vi "Set Smooth Diff Window.vi"(8 "error in (no error)":errorcluster, 10 "Window":i32=10, 11 "MF3 in":refnum<class "MF3.lvclass">) -> (0 "error out":errorcluster, 3 "MF3 out":refnum<class "MF3.lvclass">)   [LabVIEW 2011, in "MF3.lvclass"]
uses:
  MF3.lvclass
  MF3.lvclass/MF3.ctl
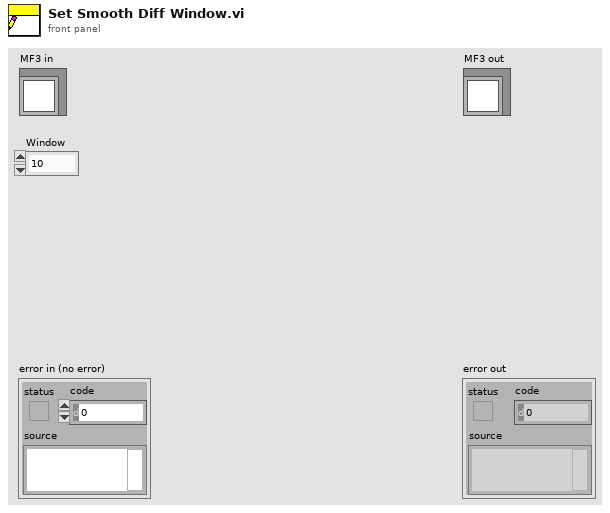
[diagram p1: front panel]
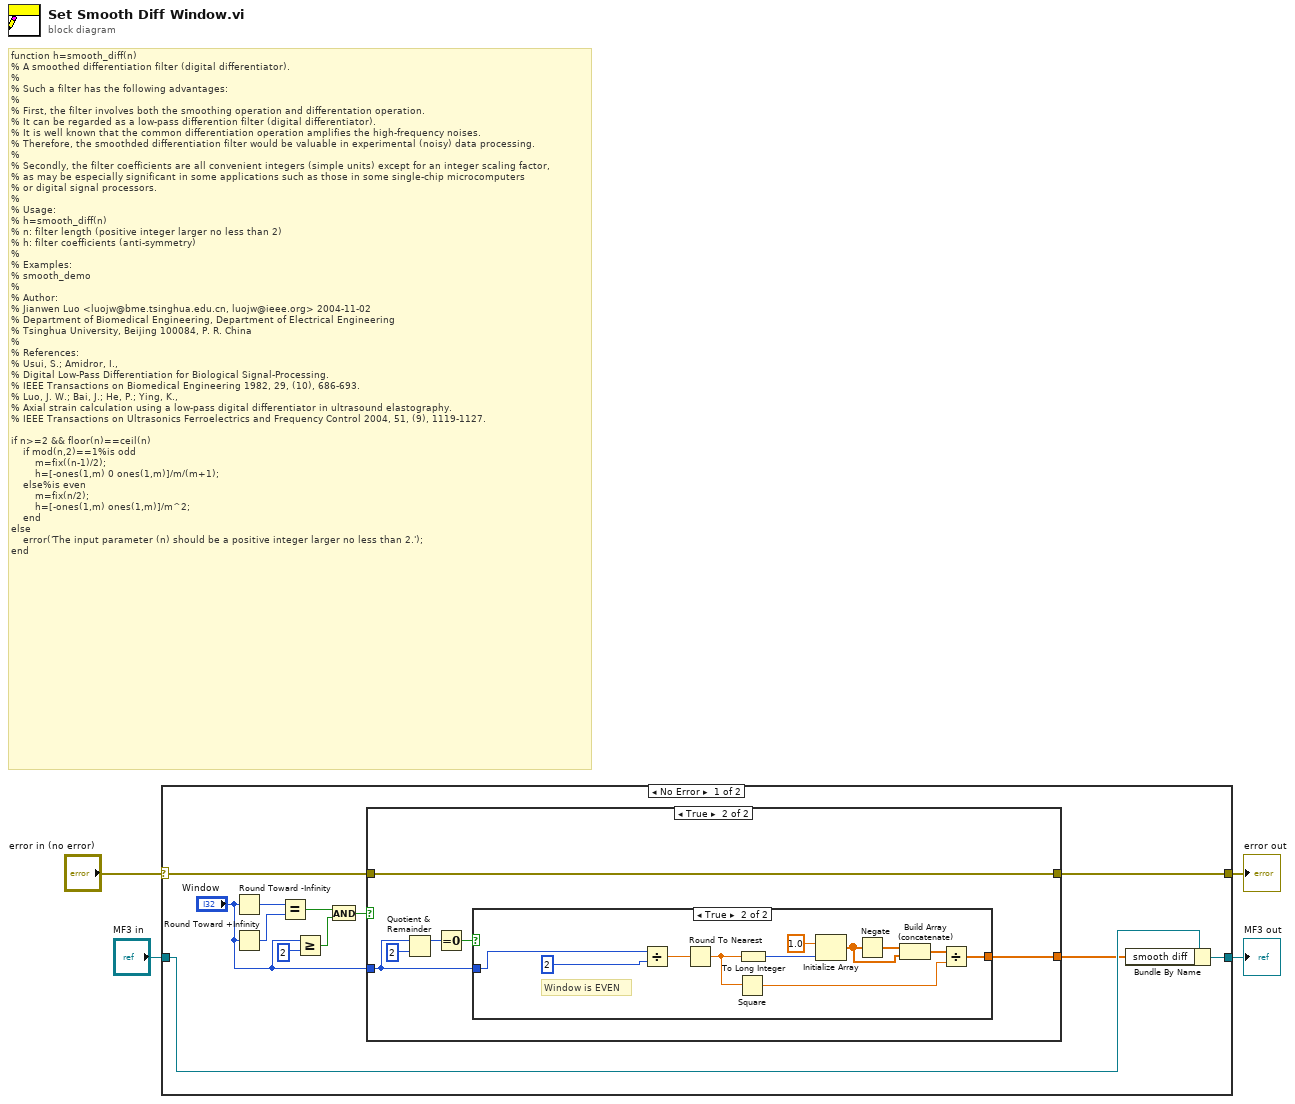
[diagram p0: block diagram]
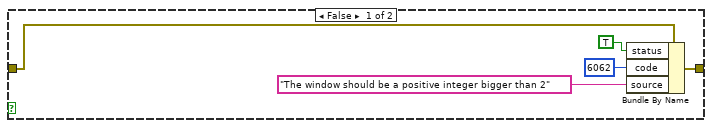
[diagram p2: hidden frame]
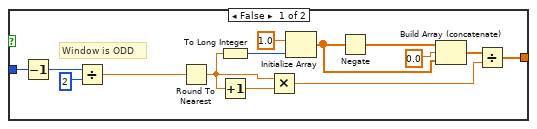
[diagram p3: hidden frame]
diagram:
  # "function h=smooth_diff(n)\n% A smoothed differentiation filter (digital differentiator). \n%\n% Such a filter has the following advantages:\n% \n% First, the filter involves both the smoothing operation and differentation operation. \n% It can be regarded as a low-pass differention filter (digital differentiator). \n% It is well known that the common differentiation operation amplifies the high-frequency noises.\n% Therefore, the smoothded differentiation filter would be valuable in experimental (noisy) data processing. \n% \n% Secondly, the filter coefficients are all convenient integers (simple units) except for an integer scaling factor,\n% as may be especially significant in some applications such as those in some single-chip microcomputers\n% or digital signal processors. \n% \n% Usage:\n% h=smooth_diff(n)\n% n: filter length (positive integer larger no less than 2)\n% h: filter coefficients (anti-symmetry)\n%\n% Examples:\n% smooth_demo\n%\n% Author:\n% Jianwen Luo <luojw@bme.tsinghua.edu.cn, luojw@ieee.org> 2004-11-02\n% Department of Biomedical Engineering, Department of Electrical Engineering\n% Tsinghua University, Beijing 100084, P. R. China  \n% \n% References:\n% Usui, S.; Amidror, I., \n% Digital Low-Pass Differentiation for Biological Signal-Processing. \n% IEEE Transactions on Biomedical Engineering 1982, 29, (10), 686-693.\n% Luo, J. W.; Bai, J.; He, P.; Ying, K., \n% Axial strain calculation using a low-pass digital differentiator in ultrasound elastography. \n% IEEE Transactions on Ultrasonics Ferroelectrics and Frequency Control 2004, 51, (9), 1119-1127.\n\nif n>=2 && floor(n)==ceil(n)\n    if mod(n,2)==1%is odd\n        m=fix((n-1)/2);\n        h=[-ones(1,m) 0 ones(1,m)]/m/(m+1);\n    else%is even\n        m=fix(n/2);\n        h=[-ones(1,m) ones(1,m)]/m^2;\n    end\nelse    \n    error('The input parameter (n) should be a positive integer larger no less than 2.');\nend"
  n1 = case shown="No Error" "error in (no error)" {
    selector: "error in (no error)" -> [w10 w53]
    tunnel: [w9 w53] -> w4
    tunnel: [w6 w54] -> w2
    tunnel: "MF3 in" -> [w7 w54]
    frame No Error {
      n2 = Round Toward -Infinity(1:"Window") -> (0:w12:i32)
      n3 = Round Toward +Infinity(x="Window") -> (ceil(x): smallest int >= x=w11:i32)
      n4 = Equal?(x=w12, y=w11) -> (x = y?=w13:bool)
      n5 = Greater Or Equal?(x="Window", y=2) -> (x >= y?=w15:bool)
      n6 = And(x=w13, y=w15) -> (x .and. y?=w16:bool)
      n7 = case shown="True" w16 {
        tunnel: [w21 w27] -> w9
        tunnel: w10 -> [w17 w27]
        tunnel: "Window" -> [_ w23]
        tunnel: [_ w22] -> w5
        frame False {
          n8 = Bundle By Name(cluster=w17, "status"=TRUE, "code"=6062, "source"="The window should be a positive integer bigger than 2") -> (w21:errorcluster)
        }
        frame True {
          n9 = Quotient & Remainder(x=w23, y=2) -> (x-y*floor(x/y)=w25:i32)  [unwired: 1 out]
          n10 = Equal To 0?(x=w25) -> (x = 0?=w24:bool)
          n11 = case shown="True" w24 {
            tunnel: w23 -> [w41 w47]
            tunnel: [w31 w45] -> w22
            frame False {
              # "Window is ODD"
              n12 = Decrement(x=w41) -> (x-1=w40:i32)
              n13 = Divide(x=w40, y=2) -> (x/y=w38:dbl)
              n14 = Round To Nearest(number=w38) -> (nearest integer value=w28:dbl)
              n15 = To Long Integer(number=w28) -> (32bit integer=w37:i32)
              n16 = Increment(x=w28) -> (x+1=w29:dbl)
              n17 = Multiply(x=w28, y=w29) -> (x*y=w30:dbl)
              n18 = Initialize Array(1.0 ("element"), w37) -> (w33:dbl[])
              n19 = Negate(x=w33) -> (-x=w35:dbl[])
              n20 = Build Array (concatenate)(w35, 0.0 ("element"), w33) -> (w32:dbl[])
              n21 = Divide(x=w32, y=w30) -> (x/y=w31:dbl[])
            }
            frame True {
              # "Window is EVEN"
              n22 = Divide(x=w47, y=2) -> (x/y=w51:dbl)
              n23 = Round To Nearest(number=w51) -> (nearest integer value=w43:dbl)
              n24 = Square(x=w43) -> (x^2=w44:dbl)
              n25 = To Long Integer(number=w43) -> (32bit integer=w50:i32)
              n26 = Initialize Array(1.0 ("element"), w50) -> (w42:dbl[])
              n27 = Negate(x=w42) -> (-x=w48:dbl[])
              n28 = Build Array (concatenate)(w48, w42) -> (w46:dbl[])
              n29 = Divide(x=w46, y=w44) -> (x/y=w45:dbl[])
            }
          }
        }
      }
      n30 = Bundle By Name(cluster=w7, "smooth diff"=w5) -> (w6:refnum<class "MF3.lvclass">)
    }
    frame Error {
    }
  }
  "error out" <- w4
  "MF3 out" <- w2
